vi "acquireValue.vi"(8 "error in (no error)":errorcluster, 10 "nextSample?":bool, 11 "performZeroCalib in":refnum<class "performZeroCalib.lvclass">) -> (0 "error out":errorcluster, 1 "function return":i32, 2 "variantData":variant, 3 "performZeroCalib out":refnum<class "performZeroCalib.lvclass">)   [LabVIEW 2016, in "SALLV_MtAtElectrometer_Messaging.lvlib" / "performZeroCalib.lvclass"]
uses:
  performZeroCalib.lvclass
  ts_sallv_MtAtElectrometer/SALLV_MtAtElectrometer.lvlib
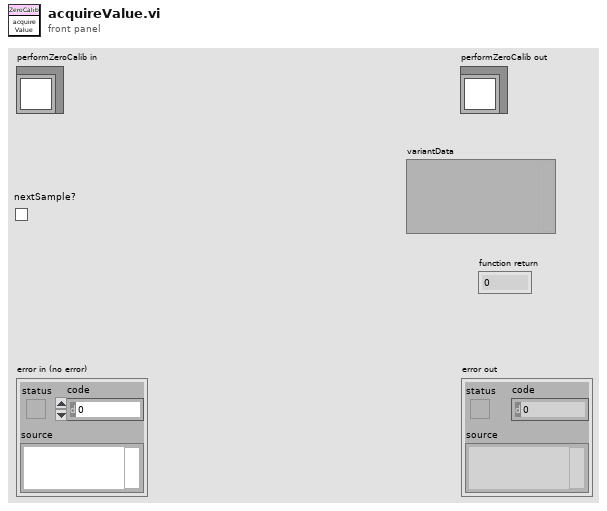
[diagram p1: front panel]
types:
  T1 = typedef "SALLV_MtAtElectrometer.lvlib/command_performZeroCalib.ctl" = cluster{"value":bool}
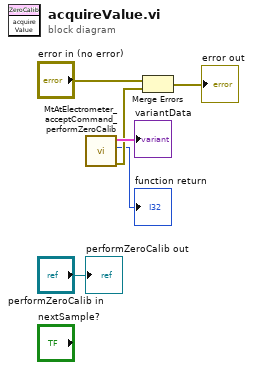
[diagram p0: block diagram]
diagram:
  n1 = call "MtAtElectrometer_acceptCommand_performZeroCalib.vi"() -> ("error out"=w2:errorcluster, "function return"=→"function return":i32, "command_performZeroCalib_Ctl out"=→"variantData":T1)  [unwired: 9 in]
  n2 = Merge Errors("error in (no error)", w2) -> (→"error out":errorcluster)
  "performZeroCalib out" <- "performZeroCalib in"
